vi "Eval y=f(a,x1,x2).vi"(5 "Variables":string[](array[string])=["x1", "x2"], 6 "number of points":u32=25, 7 "formula":string, 8 "Parameters":cluster{"name":string, "value":dbl}[](array[cluster]) {"value" format="%.2f"}, 9 "End":dbl[](array[numeric])=[1.0, 1.0] format="%.2f", 10 "Start":dbl[](array[numeric])=[0.0, 0.0] format="%.2f") -> (0 "error":i32, 1 "ticks":u32, 2 "Y Values":dbl[][](array[numeric]) format="%.2f", 3 "X2 Values":dbl[](array[numeric]) format="%.2f", 4 "X1 Values":dbl[](array[numeric]) format="%.2f")   [LabVIEW 2020, in "NI_Gmath.lvlib"]
doc: "Calculates a 2D array of function values defined on a grid."
uses:
  NI_Gmath.lvlib
panel:
  # "Example:\n\n number of points: 25 \n Start: 0.0 and 0.0\n End: 1.0 and 1.0\n Parameters: (a,1) and (b,2) \n Variables: x1 and x2\n formula: a*sin(x1)-cos(b*x2)"
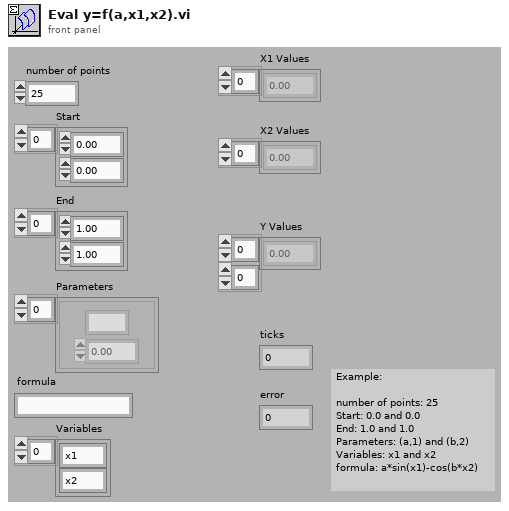
[diagram p1: front panel]
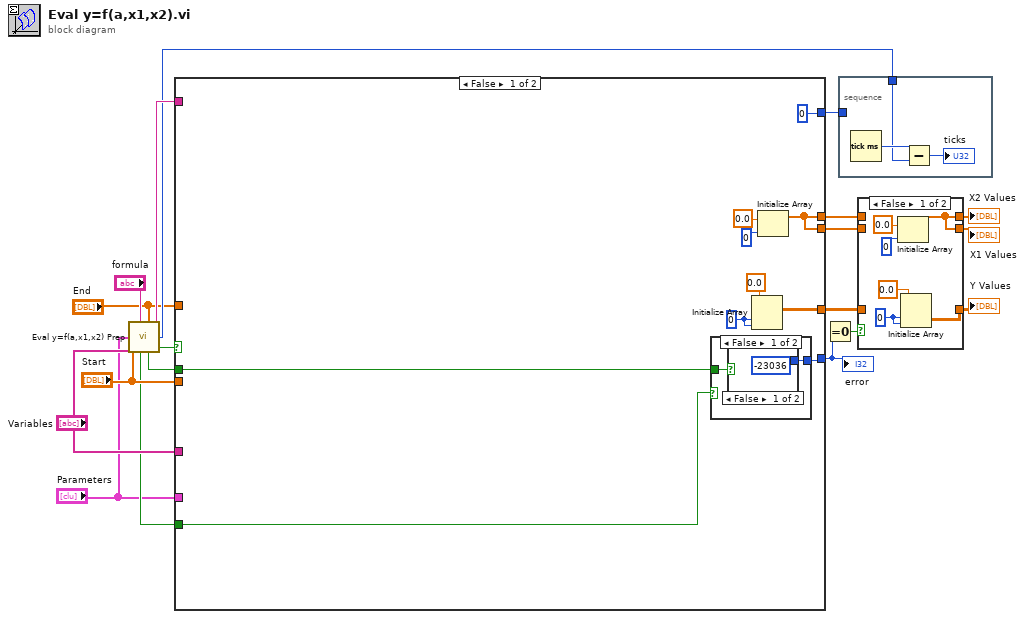
[diagram p0: block diagram]
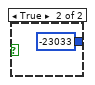
[diagram p3: hidden frame]
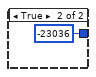
[diagram p4: hidden frame]
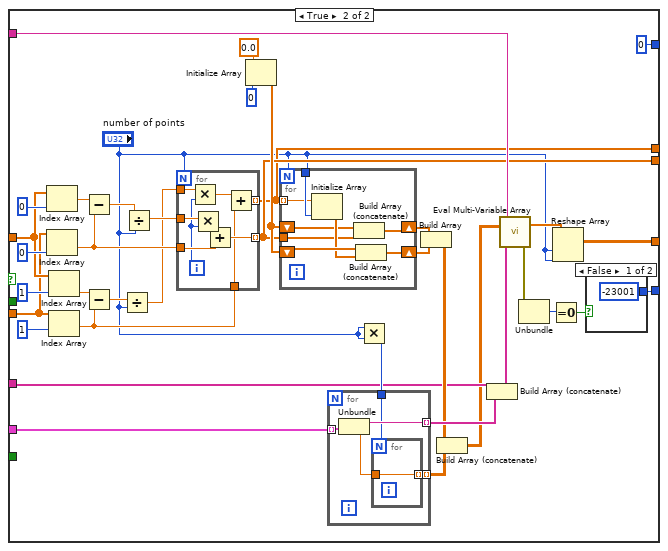
[diagram p5: hidden frame]
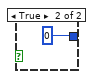
[diagram p6: hidden frame]
diagram:
  n1 = call "Eval y=f(a,x1,x2) Prep.vi"("Variables"="Variables", "formula"="formula", "Parameters"="Parameters", "Start"="Start", "End"="End") -> ("error situation 2"=w2:bool, "formula copy"=w18:string, "time [msec]"=w17:u32, "error situation 1"=w4:bool, "error (general)"=w14:bool)
  n2 = case shown="False" w14 {
    tunnel: [0 0] -> w19
    tunnel: w18 -> [_ w53]
    tunnel: "Variables" -> [_ w46]
    tunnel: [w26 w52] -> w10
    tunnel: "Parameters" -> [_ w48]
    tunnel: "End" -> [_ w43]
    tunnel: "Start" -> [_ w42]
    tunnel: [w27 w39] -> w12
    tunnel: [w23 w37] -> w7
    tunnel: [w23 w36] -> w8
    tunnel: w4 -> [w21 _]
    tunnel: w2 -> [w20 _]
    frame False {
      w28 = 0
      n3 = case shown="False" w20 {
        tunnel: w21 -> [w31 _]
        tunnel: [w30 -23036] -> w27
        frame False {
          n4 = case shown="False" w31 {
            tunnel: [-23036 -23033] -> w30
            frame False {
            }
            frame True {
            }
          }
        }
        frame True {
        }
      }
      n5 = Initialize Array(0.0, w28, w28) -> (w26:dbl[][])
      n6 = Initialize Array(0.0, 0) -> (w23:dbl[])
    }
    frame True {
      n7 = Index Array(array=w43, index=0) -> (element=w68:dbl)
      n8 = Index Array(array=w42, index=0) -> (element=w69:dbl)
      n9 = Index Array(array=w43, index=1) -> (element=w70:dbl)
      n10 = Index Array(array=w42, index=1) -> (element=w71:dbl)
      n11 = Subtract(x=w68, y=w69) -> (x-y=w54:dbl)
      n12 = Subtract(x=w70, y=w71) -> (x-y=w61:dbl)
      n13 = Divide(x=w61, y="number of points") -> (x/y=w62:dbl)
      n14 = Divide(x=w54, y="number of points") -> (x/y=w63:dbl)
      n15 = for {
        N: "number of points" -> [_]
        tunnel: w63 -> [w89]
        tunnel: w69 -> [w87]
        tunnel: [w86] -> w37 mode=indexing
        tunnel: w62 -> [w85]
        tunnel: w71 -> [w82]
        tunnel: [w81] -> w36 mode=indexing
        i -> [w84]
        n16 = Multiply(x=w85, y=w84) -> (x*y=w83:dbl)
        n17 = Multiply(x=w89, y=w84) -> (x*y=w88:dbl)
        n18 = Add(x=w88, y=w87) -> (x+y=w86:dbl)
        n19 = Add(x=w83, y=w82) -> (x+y=w81:dbl)
      }
      n20 = Initialize Array(0.0, 0) -> (w58:dbl[])
      n21 = for {
        N: "number of points" -> [_]
        tunnel: "number of points" -> [w97]
        tunnel: w36 -> [w96] mode=indexing
        shift-right: [w94] -> w60
        shift-left: w58 -> [w95]
        shift-right: [w92] -> w59
        shift-left: w58 -> [w91]
        tunnel: w37 -> [w90]
        n22 = Initialize Array(w96, w97) -> (w93:dbl[])
        n23 = Build Array (concatenate)(w91, w90) -> (w92:dbl[])
        n24 = Build Array (concatenate)(w95, w93) -> (w94:dbl[])
      }
      n25 = Multiply(x="number of points", y="number of points") -> (x*y=w49:u32)
      n26 = for {
        tunnel: w48 -> [w79] mode=indexing
        tunnel: [w78] -> w51 mode=indexing
        tunnel: w49 -> [w77]
        tunnel: [w75] -> w50 mode=indexing
        n27 = Unbundle(w79) -> ("name"=w78:string, "value"=w76:dbl)
        n28 = for {
          N: w77 -> [_]
          tunnel: [w80] -> w75 mode=indexing
          tunnel: w76 -> [w80]
        }
      }
      n29 = Build Array(w59, w60) -> (w47:dbl[][])
      n30 = Build Array (concatenate)(w47, w50) -> (w38:dbl[][])
      n31 = Build Array (concatenate)(w46, w51) -> (w44:string[])
      n32 = call "Eval Multi-Variable Array.vi"("Variables"=w44, "X Values"=w38, "formula"=w53) -> ("error out"=w45:errorcluster, "Y Values"=w55:dbl[])  [unwired: 1 in]
      n33 = Unbundle(w45) -> ("code"=w40:i32)  [unwired: 2 out]
      n34 = Equal To 0?(x=w40) -> (x = 0?=w41:bool)
      n35 = Reshape Array(w55, "number of points", "number of points") -> (w52:dbl[][])
      n36 = case shown="False" w41 {
        tunnel: [-23001 0] -> w39
        frame False {
        }
        frame True {
        }
      }
    }
  }
  "error" <- w12
  n37 = Equal To 0?(x=w12) -> (x = 0?=w11:bool)
  n38 = stacked-sequence {
    tunnel: w19 -> [_]
    tunnel: w17 -> [w98]
    frame #0 {
      n39 = Tick Count (ms)() -> (millisecond timer value=w100:u32)
      n40 = Subtract(x=w100, y=w98) -> (x-y=→"ticks":u32)
    }
  }
  n41 = case shown="False" w11 {
    tunnel: w10 -> [_ w109]
    tunnel: [w104 w109] -> w9
    tunnel: w8 -> [_ w108]
    tunnel: [w101 w108] -> w6
    tunnel: w7 -> [_ w107]
    tunnel: [w101 w107] -> w5
    frame False {
      w106 = 0
      n42 = Initialize Array(0.0, 0) -> (w101:dbl[])
      n43 = Initialize Array(0.0, w106, w106) -> (w104:dbl[][])
    }
    frame True {
    }
  }
  "Y Values" <- w9
  "X1 Values" <- w5
  "X2 Values" <- w6
